vi "密码比对.vi"(8 "密码":string, 9 "账户":string, 11 "文件（使用对话框）":path) -> (1 "x = y?":bool)   [LabVIEW 2015]
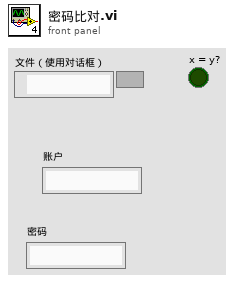
[diagram p1: front panel]
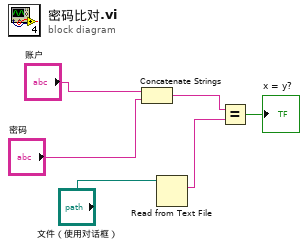
[diagram p0: block diagram]
diagram:
  n1 = Concatenate Strings("账户", "密码") -> (w4:string)
  n2 = Read from Text File(file (use dialog)="文件（使用对话框）") -> (text=w3:string)  [unwired: 3 in, 3 out]
  n3 = Equal?(x=w4, y=w3) -> (x = y?=→"x = y?":bool)
